vi "EnumCaseString.vi"(5 "selector string":string, 8 "data type":variant) -> (1 "Default":bool, 4 "case":string)   [LabVIEW 2014, in "CaseStructure.lvclass"]
uses:
  CaseStructure.lvclass
  Python/Parsing/ListTypesTD.ctl
  <vilib>/regexp/Match Regular Expression.xnode
  Python/Parsing/Python Functions.lvlib
  <vilib>/Utility/VariantDataType/VariantType.lvlib
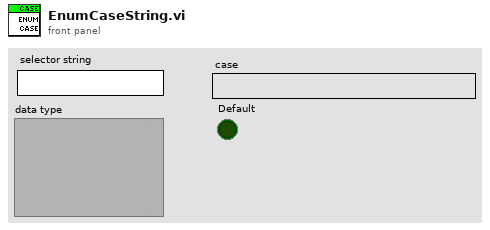
[diagram p1: front panel]
types:
  T1 = typedef "Python Functions.lvlib/ListTypesTD.ctl" = enum16{"list", "tuple", "parameter list", "output list", "return values"}
  T2 = typedef "VariantType.lvlib/Type.ctl" = enum8{"Invalid Type", "Void", "I8", "I16", "I32", "I64", "U8", "U16", "U32", "U64", "Single Float", "Double Float", "Extended Float", "Single Complex", "Double Complex", "Extended Complex", "Enum U8", "Enum U16", "Enum U32", "Enum U64", "Single Float With Unit", "Double Float With Unit", "Extended Float With Unit", "Single Complex with Unit", "Double Complex with Unit", "Extended Complex with Unit", "Boolean", "String", "Path", "Picture", "Tag", "Array", "Cluster", "Variant", "LV Variant", "Waveform", "Timestamp", "Digital Waveform", "Digital Data", "ExpressData", "Refnum", "External Data", "VI", "Poly VI", "LabVIEW Class Instance", "Fixed Point"}
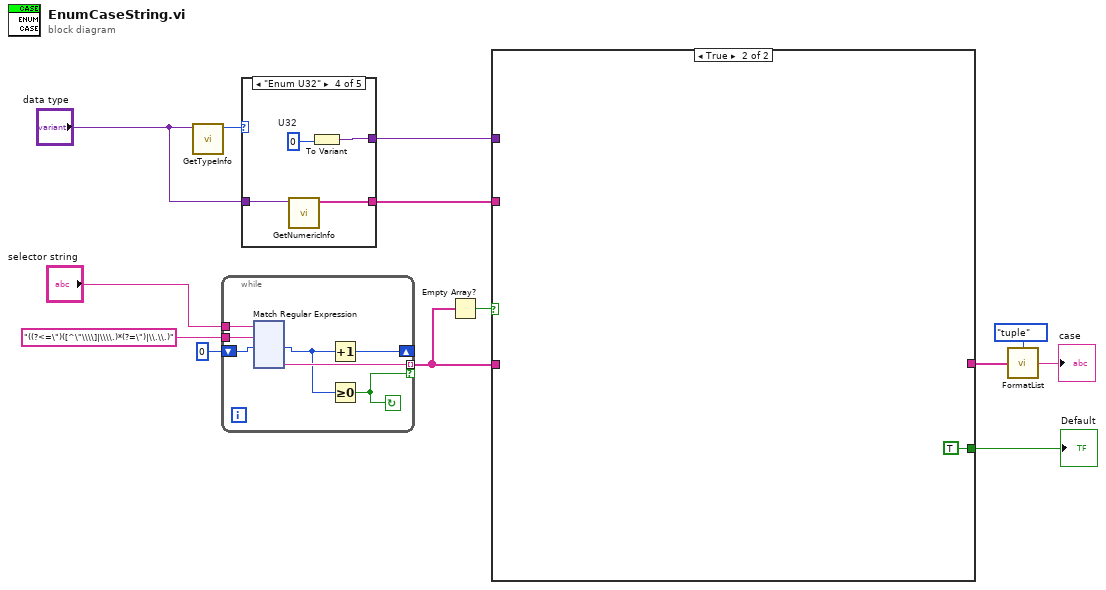
[diagram p0: block diagram]
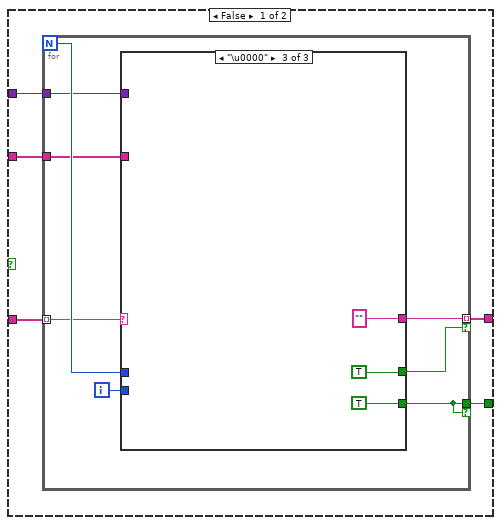
[diagram p2: hidden frame]
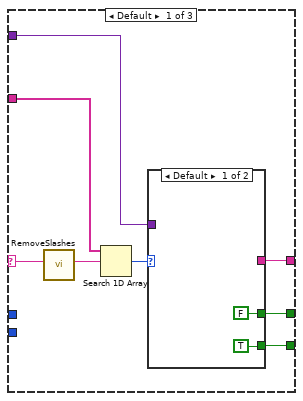
[diagram p3: hidden frame]
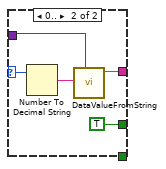
[diagram p4: hidden frame]
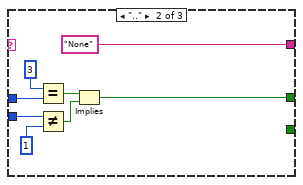
[diagram p5: hidden frame]
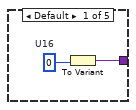
[diagram p6: hidden frame]
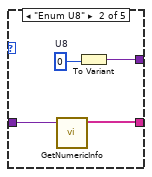
[diagram p7: hidden frame]
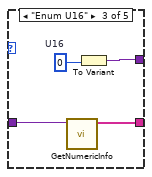
[diagram p8: hidden frame]
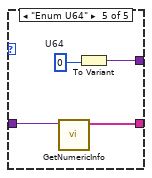
[diagram p9: hidden frame]
diagram:
  n1 = call <vilib>:"GetTypeInfo.vi"("Variant"="data type") -> ("Type Enum"=w6:T2)  [unwired: 6 in, 4 out]
  n2 = while {
    tunnel: "selector string" -> [w20]
    tunnel: "((?<=\")([^\"\\\\]|\\\\.)*(?=\")|\\.\\.)" ("regular expression") -> [w19]
    tunnel: [w17] -> w1 mode=indexing if=w16
    shift-right: [w14] -> _
    shift-left: 0 -> [w18]
    stop <- w16 continue-if-true
    n3 = xnode "Match Regular Expression"("input string"=w20, "regular expression"=w19, "offset (0)"=w18) -> ("offset past match"=w15:i32, "submatch 1"=w17:string)  [unwired: 3 in, 4 out]
    n4 = Increment(x=w15) -> (x+1=w14:i32)
    n5 = Greater Or Equal To 0?(x=w15) -> (x >= 0?=w16:bool)
  }
  n6 = case shown="\"Enum U32\"" w6 {
    tunnel: [w134 w138 w142 w146 w150] -> w5
    tunnel: "data type" -> [_ w137 w141 w145 w149]
    tunnel: [_ w136 w140 w144 w148] -> w3
    frame Default {
      w135 = u16 0  # U16
      n7 = To Variant(anything=w135) -> (Variant=w134:variant)
    }
    frame "Enum U8" {
      w139 = u8 0  # U8
      n8 = call <vilib>:"GetNumericInfo.vi"("Variant"=w137) -> ("EnumNames"=w136:string[])  [unwired: 7 in, 3 out]
      n9 = To Variant(anything=w139) -> (Variant=w138:variant)
    }
    frame "Enum U16" {
      w143 = u16 0  # U16
      n10 = call <vilib>:"GetNumericInfo.vi"("Variant"=w141) -> ("EnumNames"=w140:string[])  [unwired: 7 in, 3 out]
      n11 = To Variant(anything=w143) -> (Variant=w142:variant)
    }
    frame "Enum U32" {
      w147 = u32 0  # U32
      n12 = call <vilib>:"GetNumericInfo.vi"("Variant"=w145) -> ("EnumNames"=w144:string[])  [unwired: 7 in, 3 out]
      n13 = To Variant(anything=w147) -> (Variant=w146:variant)
    }
    frame "Enum U64" {
      w151 = u64 0  # U64
      n14 = call <vilib>:"GetNumericInfo.vi"("Variant"=w149) -> ("EnumNames"=w148:string[])  [unwired: 7 in, 3 out]
      n15 = To Variant(anything=w151) -> (Variant=w150:variant)
    }
  }
  n16 = Empty Array?(array=w1) -> (empty?=w2:bool)
  n17 = case shown="True" w2 {
    tunnel: w1 -> [w156 _]
    tunnel: [w155 _] -> w9
    tunnel: [w154 TRUE] -> w8
    tunnel: w5 -> [w153 _]
    tunnel: w3 -> [w152 _]
    frame False {
      n18 = for {
        N -> [w164]
        tunnel: w156 -> [w163] mode=indexing
        tunnel: [w162] -> w155 mode=indexing if=w159
        tunnel: [w161] -> w154 if=w161
        tunnel: w153 -> [w158]
        tunnel: w152 -> [w157]
        i -> [w160]
        n19 = case shown="\"\"" w163 {
          selector: w163 -> [w171 _ _]
          tunnel: [w172 "None" "" ("value")] -> w162
          tunnel: [w165 _ TRUE] -> w161
          tunnel: w160 -> [_ w186 _]
          tunnel: w164 -> [_ w184 _]
          tunnel: [w166 w182 TRUE] -> w159
          tunnel: w158 -> [w170 _ _]
          tunnel: w157 -> [w168 _ _]
          frame Default {
            n20 = call "RemoveSlashes.vi"("slashed string"=w171) -> ("unslashed"=w169:string)  [unwired: 10 in]
            n21 = Search 1D Array(1D array=w168, element=w169) -> (index of element=w167:i32)  [unwired: 1 in]
            n22 = case shown="Default" w167 {
              selector: w167 -> [_ w177]
              tunnel: [_ w179] -> w172
              tunnel: w170 -> [_ w178]
              tunnel: [FALSE TRUE] -> w166
              tunnel: [TRUE _] -> w165
              frame Default {
              }
              frame 0.. {
                n23 = Number To Decimal String(number=w177) -> (decimal integer string=w176:string)  [unwired: 1 in]
                n24 = call "DataValueFromString.vi"("Type"=w178, "value"=w176) -> ("value"=w179:string)  [unwired: 7 in]
              }
            }
          }
          frame ".." {
            n25 = Equal?(x=3, y=w184) -> (x = y?=w181:bool)
            n26 = Not Equal?(x=w186, y=1) -> (x != y?=w180:bool)
            n27 = Implies(1:w180, 2:w181) -> (0:w182:bool)
          }
          frame "\u0000" {
          }
        }
      }
    }
    frame True {
    }
  }
  "Default" <- w8
  n28 = call "FormatList.vi"("values"=w9, "type"=ListTypesTD."tuple") -> ("python object"=→"case":string)
